vi "test_relay.vi"() -> ()   [LabVIEW 2019]
panel:
  out "bits_set":i32
  out "ch_2_out":bool
  out "ch_1_out":bool
  out "ch_2_set":bool
  out "ch_1_set":bool
  out "time":timestamp format="%<%Y-%m-%d %H:%M:%S>T"
  out "status":bool
  in  "wait (ms)":u32=2000
  in  "stop":bool
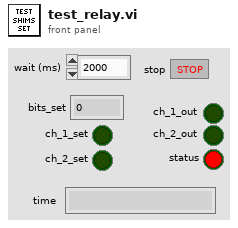
[diagram p1: front panel]
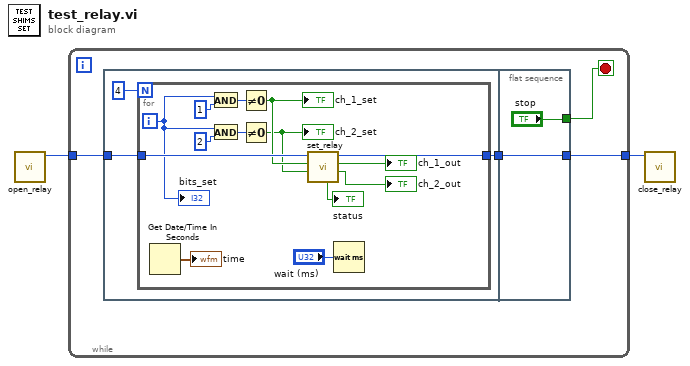
[diagram p0: block diagram]
diagram:
  n1 = call "open_relay.vi"() -> ("Handle"=w2:u64)  [unwired: 8 in, 3 out]
  n2 = while {
    tunnel: w2 -> [w6]
    tunnel: [w5] -> w1
    stop <- w3 stop-if-true
    n3 = flat-sequence {
      tunnel: w6 -> [w8]
      tunnel: [w7] -> w4
      tunnel: [w25] -> w5
      tunnel: w4 -> [w25]
      tunnel: ["stop"] -> w3
      frame #0 {
        n4 = for {
          N: 4 -> [_]
          tunnel: w8 -> [w21]
          tunnel: [w20] -> w7
          i -> [w15]
          n5 = Get Date/Time In Seconds() -> (seconds since 1Jan1904=→"time":timestamp)
          n6 = And(x=w15, y=u32 1) -> (x .and. y?=w18:u32)
          n7 = And(x=w15, y=u32 2) -> (x .and. y?=w16:u32)
          n8 = Not Equal To 0?(x=w18) -> (x != 0?=w14:bool)
          "ch_1_set" <- w14
          n9 = Not Equal To 0?(x=w16) -> (x != 0?=w13:bool)
          "ch_2_set" <- w13
          n10 = call "set_relay.vi"("ch_2"=w13, "ch_1"=w14, "Handle"=w21) -> ("ch_2_out"=→"ch_2_out":bool, "ch_1_out"=→"ch_1_out":bool, "Handle_out"=w20:u64, "status"=→"status":bool)  [unwired: 4 in, 1 out]
          n11 = Wait (ms)(milliseconds to wait="wait (ms)") -> ()  [unwired: 1 out]
          "bits_set" <- w15
        }
      }
      frame #1 {
      }
    }
  }
  n12 = call "close_relay.vi"("Handle"=w1) -> ()  [unwired: 9 in, 2 out]
